vi "RFConfig_SubVI_HMCT22##_SettingConfiguration.vi"(7 "Apply Configurations":bool, 8 "error in (no error)":errorcluster, 9 "Frequency (GHz)":dbl format="%#_12g", 10 "Power (dBm)":dbl, 11 "VISA Refnum in":refnum<visa-resource-name>) -> (0 "error out":errorcluster, 1 "Frequency (GHz) Output":dbl, 2 "Power (dBm) Output":dbl)   [LabVIEW 2019]
panel:
  out "Power (dBm)":string
  out "frequency (GHz)":string
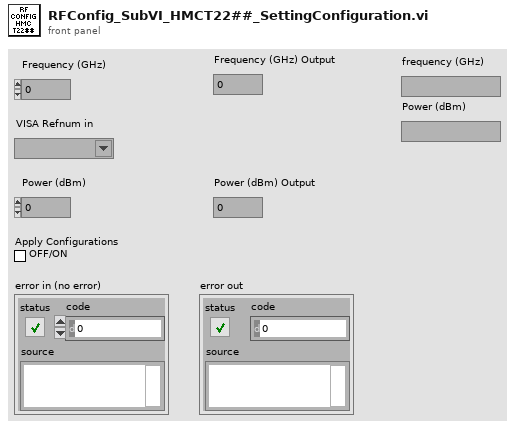
[diagram p1: front panel]
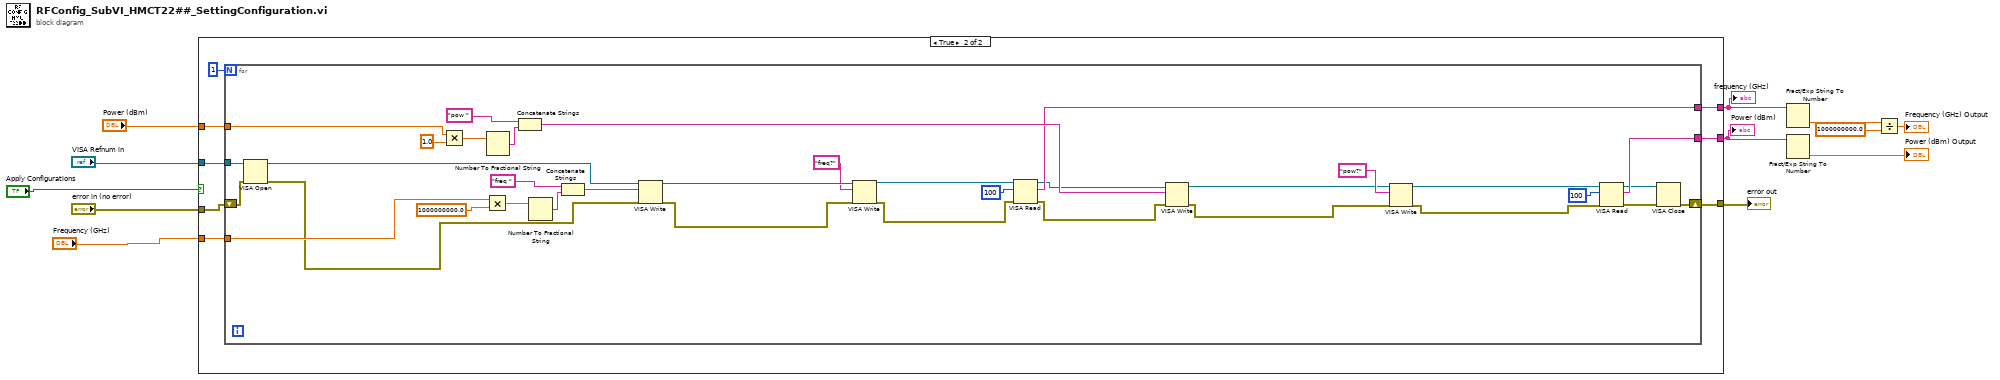
[diagram p0: block diagram]
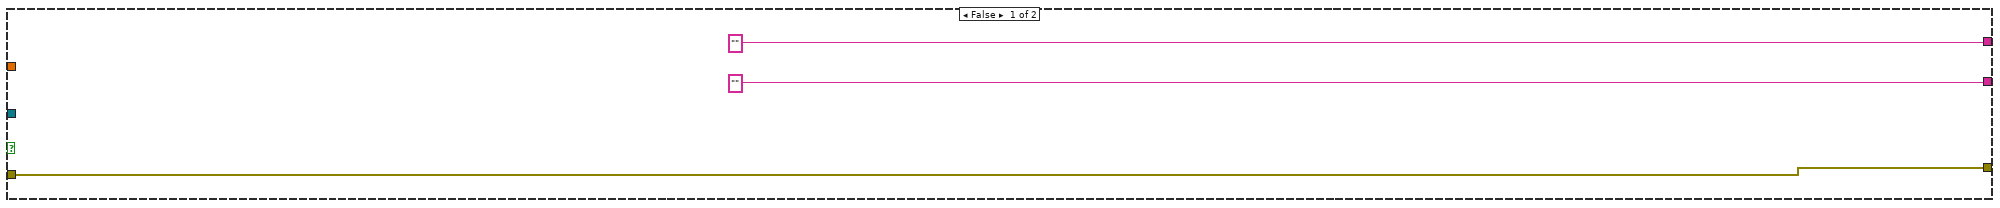
[diagram p2: hidden frame]
diagram:
  n1 = case shown="True" "Apply Configurations" {
    tunnel: [w15 w23] -> w8
    tunnel: "error in (no error)" -> [w15 w22]
    tunnel: "VISA Refnum in" -> [_ w21]
    tunnel: "Frequency (GHz)" -> [_ w20]
    tunnel: "Power (dBm)" -> [_ w19]
    tunnel: ["" ("read buffer") w18] -> w6
    tunnel: ["" ("read buffer") w17] -> w5
    frame False {
    }
    frame True {
      n2 = for {
        N: 1 -> [_]
        tunnel: w21 -> [w45]
        tunnel: w20 -> [w44]
        tunnel: w19 -> [w43]
        tunnel: [w38] -> w18
        tunnel: [w32] -> w17
        shift-right: [w58] -> w23
        shift-left: w22 -> [w57]
        n3 = VISA Open(error in (no error)=w57, VISA resource name=w45) -> (VISA resource name=w51:refnum<visa-resource-name>, error out=w24:errorcluster)  [unwired: 3 in]
        n4 = Multiply(x=w43, y=1.0) -> (x*y=w49:dbl)
        n5 = Multiply(x=w44, y=1000000000.0) -> (x*y=w55:dbl)
        n6 = Number To Fractional String(number=w49) -> (F-format string=w50:string)  [unwired: 3 in]
        n7 = Concatenate Strings("pow " ("string"), w50) -> (w46:string)
        n8 = Number To Fractional String(number=w55) -> (F-format string=w56:string)  [unwired: 3 in]
        n9 = Concatenate Strings("freq " ("string"), w56) -> (w54:string)
        n10 = VISA Write(VISA resource name=w51, write buffer=w54, error in (no error)=w24) -> (VISA resource name out=w40:refnum<visa-resource-name>, error out=w25:errorcluster)  [unwired: 1 out]
        n11 = VISA Write(VISA resource name=w40, write buffer="freq?", error in (no error)=w25) -> (VISA resource name out=w41:refnum<visa-resource-name>, error out=w26:errorcluster)  [unwired: 1 out]
        n12 = VISA Read(VISA resource name=w41, byte count=u32 100, error in (no error)=w26) -> (VISA resource name out=w34:refnum<visa-resource-name>, read buffer=w38:string, error out=w27:errorcluster)  [unwired: 1 out]
        n13 = VISA Write(VISA resource name=w34, write buffer=w46, error in (no error)=w27) -> (VISA resource name out=w33:refnum<visa-resource-name>, error out=w28:errorcluster)  [unwired: 1 out]
        n14 = VISA Write(VISA resource name=w33, write buffer="pow?", error in (no error)=w28) -> (VISA resource name out=w36:refnum<visa-resource-name>, error out=w29:errorcluster)  [unwired: 1 out]
        n15 = VISA Read(VISA resource name=w36, byte count=u32 100, error in (no error)=w29) -> (VISA resource name out=w31:refnum<visa-resource-name>, read buffer=w32:string, error out=w30:errorcluster)  [unwired: 1 out]
        n16 = VISA Close(VISA resource name=w31, error in (no error)=w30) -> (error out=w58:errorcluster)
      }
    }
  }
  "error out" <- w8
  "frequency (GHz)" <- w6
  "Power (dBm)" <- w5
  n17 = Fract/Exp String To Number(string=w6) -> (number=w3:dbl)  [unwired: 3 in, 1 out]
  n18 = Fract/Exp String To Number(string=w5) -> (number=→"Power (dBm) Output":dbl)  [unwired: 3 in, 1 out]
  n19 = Divide(x=w3, y=1000000000.0) -> (x/y=→"Frequency (GHz) Output":dbl)
